vi "Handle Subscription Requests.vi"(7 "subscriptions queue":refnum<queue>, 8 "error in":errorcluster, 9 "sub map":refnum<data-value>, 10 "nats connection in":T1={"connection ID"=refnum, "server INFO"="", "timeout ms"=5000, "verbose?"=FALSE, "server headers?"=FALSE, "client headers?"=FALSE}, 11 "subs in":T2) -> (0 "error out":errorcluster, 3 "subs out":T2)   [LabVIEW 2024, in "NATS Client.lvlib" / "NATS Client.lvclass"]
uses:
  NATS Client.lvclass
  Subscription Map.ctl
  NATS Subscription/NATS Subscription.lvclass
  subscription queue.ctl
  subscription actions.ctl
  <vilib>/NATS/NATS Core/Controls/nats connection.ctl
  NATS Subscription/NATS Subscription.lvclass/NATS Subscription.ctl
  NATS Subscription/get id.vi
  NATS Subscription/get subject.vi
  NATS Subscription/Get queue.vi
  <vilib>/dlg_ctls.llb/Space Constant.vi
  <vilib>/NATS/NATS Core/VIs/subVIs/Set Timeout.vi
  NATS Client.lvclass/NATS Client.ctl
  <vilib>/NATS/NATS Core/NATS Core.lvlib
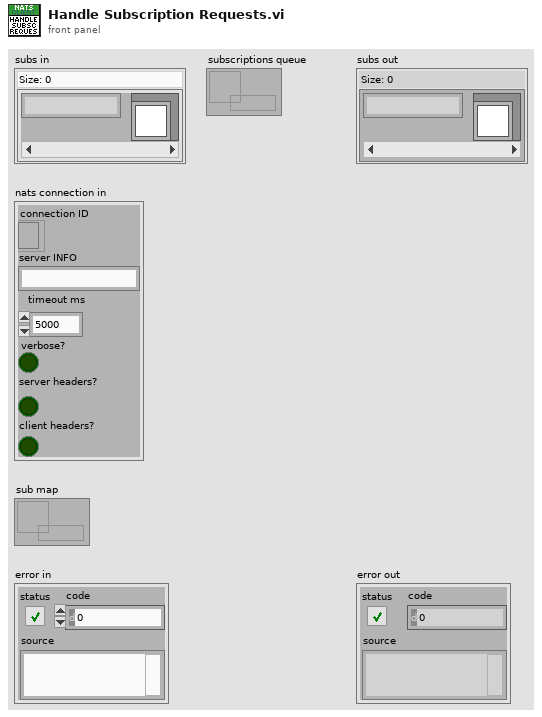
[diagram p1: front panel]
types:
  T1 = typedef "NATS Core.lvlib/nats connection.ctl" = cluster{"connection ID":refnum<k5>, "server INFO":string, "timeout ms":i32, "verbose?":bool, "server headers?":bool, "client headers?":bool}
  T2 = typedef "NATS Client.lvlib/NATS Client.lvclass/Subscription Map.ctl" = map{string, refnum<class "NATS Subscription.lvclass">}
  T3 = typedef "NATS Client.lvlib/NATS Client.lvclass/subscription queue.ctl" = cluster{"action":T4, "subscription":refnum<class "NATS Subscription.lvclass">}
  T4 = typedef "NATS Client.lvlib/NATS Client.lvclass/subscription actions.ctl" = enum16{"sub", "unsub"}
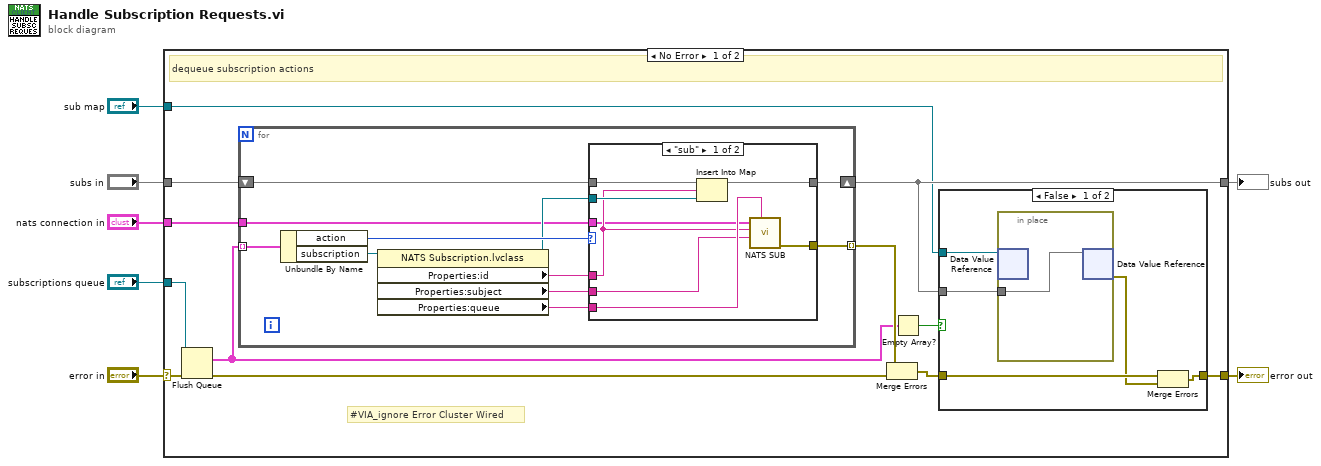
[diagram p0: block diagram]
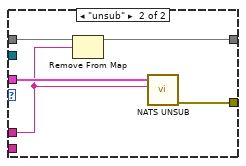
[diagram p3: hidden frame]
diagram:
  n1 = case shown="No Error" "error in" {
    selector: "error in" -> [w11 w51]
    tunnel: "subs in" -> [w19 w52]
    tunnel: [w18 w52] -> w6
    tunnel: [w16 w51] -> w7
    tunnel: "sub map" -> [w17 _]
    tunnel: "nats connection in" -> [w14 _]
    tunnel: "subscriptions queue" -> [w10 _]
    frame No Error {
      # "#VIA_ignore Error Cluster Wired"
      # "dequeue subscription actions"
      n2 = Flush Queue(queue=w10, error in (no error)=w11) -> (remaining elements=w8:T3[], error out=w9:errorcluster)  [unwired: 1 out]
      n3 = for {
        tunnel: w8 -> [w31] mode=indexing
        shift-right: [w36] -> w18
        shift-left: w19 -> [w37]
        tunnel: w14 -> [w30]
        tunnel: [w29] -> w12 mode=indexing
        n4 = Unbundle By Name(w31) -> ("action"=w33:T4, "subscription"=w34:refnum<class "NATS Subscription.lvclass">)
        n5 = property class="NATS Subscription.lvclass"(reference=w34) -> (reference out=w32:refnum<class "NATS Subscription.lvclass">, "Properties:id"=w35:string, "Properties:subject"=w27:string, "Properties:queue"=w28:string)  [unwired: 1 in, 1 out]
        n6 = case shown="\"sub\"" w33 {
          tunnel: w37 -> [w45 w49]
          tunnel: [w44 w50] -> w36
          tunnel: w35 -> [w40 w47]
          tunnel: w32 -> [w43 _]
          tunnel: w30 -> [w38 w48]
          tunnel: [w42 w46] -> w29
          tunnel: w28 -> [w41 _]
          tunnel: w27 -> [w39 _]
          frame "sub" {
            n7 = Insert Into Map(map in=w45, key=w40, value=w43) -> (map out=w44:T2)  [unwired: 2 out]
            n8 = call <vilib>:"NATS SUB.vi"("queue group"=w41, "subject"=w39, "sub id"=w40, "nats connection in"=w38) -> ("error out"=w42:errorcluster)  [unwired: 5 in, 2 out]
          }
          frame "unsub" {
            n9 = Remove From Map(10:w47, 11:w49) -> (3:w50:T2)  [unwired: 2 out]
            n10 = call <vilib>:"NATS UNSUB.vi"("sub id"=w47, "nats connection in"=w48) -> ("error out"=w46:errorcluster)  [unwired: 8 in, 1 out]
          }
        }
      }
      n11 = Merge Errors(w12, w9) -> (w13:errorcluster)
      n12 = Empty Array?(array=w8) -> (empty?=w15:bool)
      n13 = case shown="False" w15 {
        tunnel: w13 -> [w24 w26]
        tunnel: w18 -> [w23 _]
        tunnel: w17 -> [w22 _]
        tunnel: [w21 w26] -> w16
        frame False {
          n14 = in-place {
            in-place-border: w23 -> [w25]
            n15 = in-place-dvr #1(w22) -> ()  [unwired: 2 out]
            n16 = in-place-dvr #1(w25) -> (w20:errorcluster)  [unwired: 1 out]
          }
          n17 = Merge Errors(w24, w20) -> (w21:errorcluster)
        }
        frame True {
        }
      }
    }
    frame Error {
    }
  }
  "error out" <- w7
  "subs out" <- w6
